vi "Create FP Item.vi"(6 "Cluster Component":bool, 8 "error in (no error)":errorcluster, 10 "GObject In":refnum<vi>, 11 "GCluster in":refnum<class "Cluster.lvclass">) -> (0 "error out":errorcluster, 1 "Is Control":bool, 2 "Is Indicator":bool, 3 "GCluster out":refnum<class "Cluster.lvclass">, 4 "All Objects Created":refnum<class "Object.lvclass">[](array[class]), 5 "Is Visible":bool)   [LabVIEW 2017, in "Front Panel Publisher.lvlib" / "Cluster.lvclass"]
uses:
  Cluster.lvclass
  Web Front Panel_class/Web Front Panel.lvclass
  Object_class/Object.lvclass
  Control_class/Control.lvclass
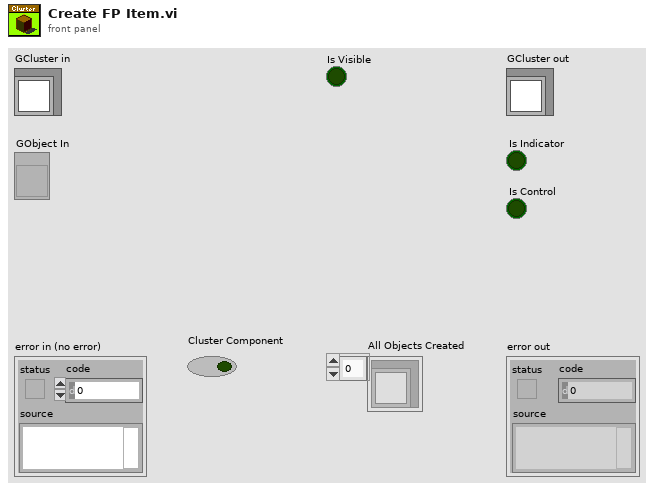
[diagram p1: front panel]
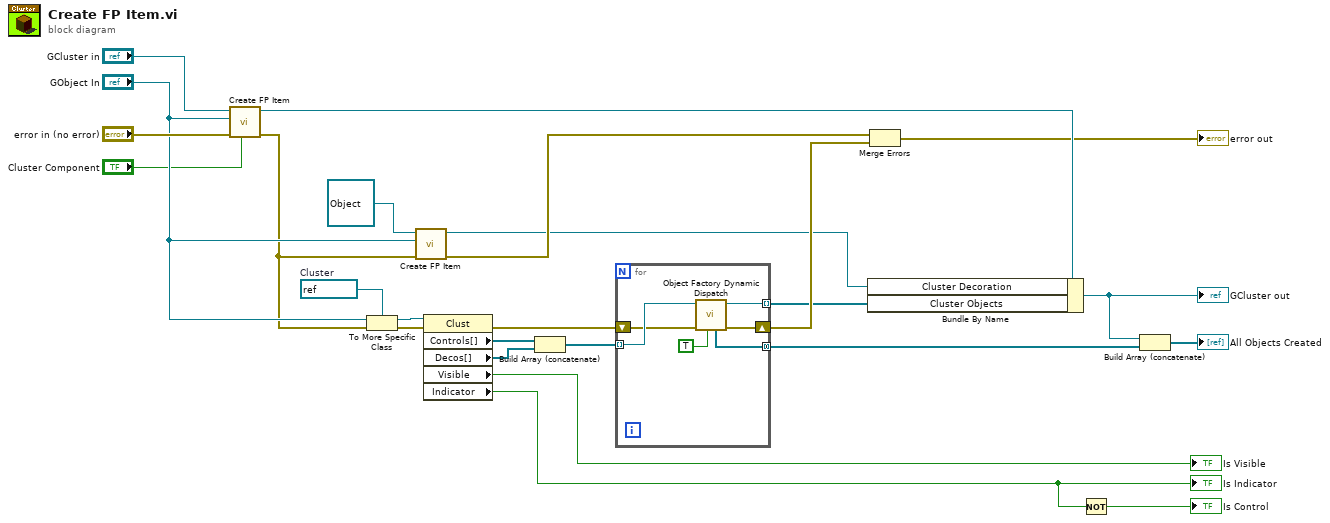
[diagram p0: block diagram]
diagram:
  w22 = refnum<vi> refnum  # Cluster
  n1 = call-parent "Create FP Item.vi"("Cluster Component"="Cluster Component", "error in (no error)"="error in (no error)", "GObject In"="GObject In", "GControl in"="GCluster in") -> ("error out"=w10:errorcluster, "GControl out"=w23:refnum<class "Cluster.lvclass">)  [unwired: 2 in, 4 out]
  n2 = To More Specific Class(target class=w22, reference="GObject In", error in=w10) -> (specific class reference=w21:refnum<vi>, error out=w20:errorcluster)
  n3 = call-dynamic "Create FP Item.vi"("error in (no error)"=w10, "GObject In"="GObject In", "GObject in"=refnum<class "Object.lvclass"> refnum) -> ("error out"=w8:errorcluster, "GObject out"=w3:refnum<class "Object.lvclass">)  [unwired: 3 in, 4 out]
  n4 = property class="Clust"(reference=w21, error in=w20) -> (error out=w18:errorcluster, "Controls[]"=w19:refnum<vi>[], "Decos[]"=w16:refnum<vi>[], "Visible"=→"Is Visible":bool, "Indicator"=w12:bool)  [unwired: 1 out]
  "Is Indicator" <- w12
  n5 = Build Array (concatenate)(w19, w16) -> (w17:refnum<vi>[])
  n6 = for {
    tunnel: w17 -> [w31] mode=indexing
    shift-right: [w29] -> w7
    shift-left: w18 -> [w30]
    tunnel: [w28] -> w6 mode=indexing
    tunnel: [w27] -> w5 mode=concatenating
    n7 = call "Object Factory Dynamic Dispatch.vi"("Cluster Component"=TRUE, "error in (no error)"=w30, "GOject In"=w31) -> ("error out"=w29:errorcluster, "Object Out"=w28:refnum<class "Object.lvclass">, "All Objects Created"=w27:refnum<class "Object.lvclass">[])  [unwired: 3 in, 3 out]
  }
  n8 = Bundle By Name(cluster=w23, "Cluster Decoration"=w3, "Cluster Objects"=w6) -> (w2:refnum<class "Cluster.lvclass">)
  "GCluster out" <- w2
  n9 = Merge Errors(w8, w7) -> (→"error out":errorcluster)
  n10 = Not(x=w12) -> (.not. x?=→"Is Control":bool)
  n11 = Build Array (concatenate)(w2, w5) -> (→"All Objects Created":refnum<class "Object.lvclass">[])
